vi "control-table.build.vi"(8 "error in (no error)":errorcluster, 11 "vi ref":refnum<vi>) -> (0 "error out":errorcluster, 3 "control table":string[][](array[string]), 5 "headers":string[](array[string])=["Label", "Caption", "Description", "Tip Strip"], 7 "control indicies":i32[](array[numeric]))   [LabVIEW 2020]
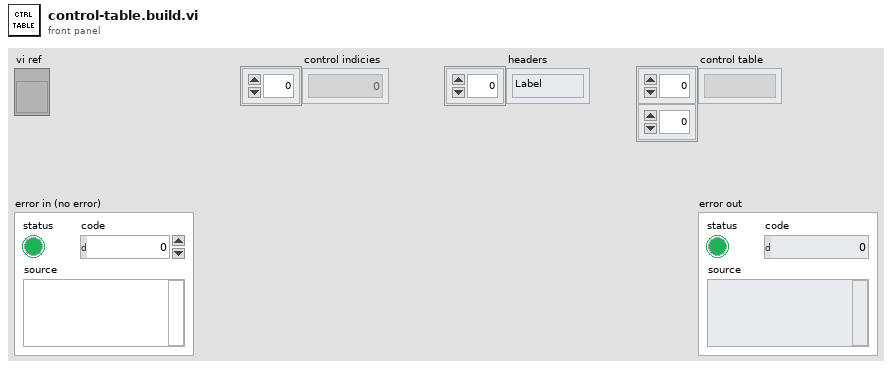
[diagram p1: front panel]
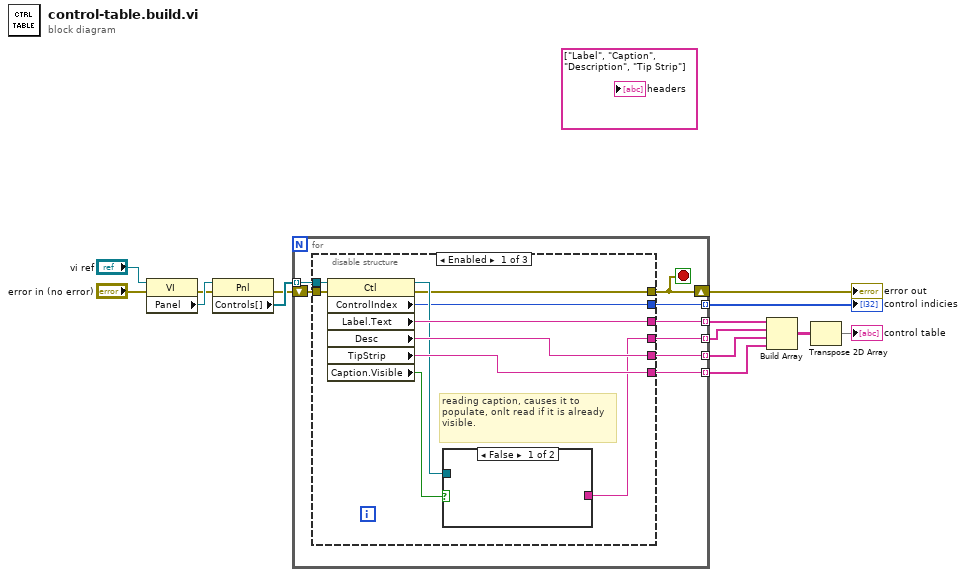
[diagram p0: block diagram]
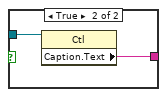
[diagram p2: hidden frame]
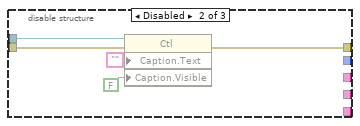
[diagram p3: hidden frame]
diagram:
  n1 = property class="VI"(reference="vi ref", error in="error in (no error)") -> (error out=w14:errorcluster, "Panel"=w15:refnum<vi>)  [unwired: 1 out]
  n2 = property class="Pnl"(reference=w15, error in=w14) -> (error out=w7:errorcluster, "Controls[]"=w13:refnum<vi>[])  [unwired: 1 out]
  n3 = for {
    tunnel: w13 -> [w23] mode=indexing
    tunnel: [w22] -> w12 mode=indexing
    tunnel: [w21] -> w11 mode=indexing
    tunnel: [w20] -> w10 mode=indexing
    tunnel: [w19] -> w8 mode=indexing
    shift-right: [w17] -> w2
    shift-left: w7 -> [w18]
    tunnel: [w16] -> w1 mode=indexing
    stop <- w17 stop-if-true
    n4 = disable-structure shown="Enabled" {
      disable-tunnel: w23 -> [w33 w40 _]
      disable-tunnel: [w32 _ _] -> w22
      disable-tunnel: [w31 _ _] -> w21
      disable-tunnel: [w30 _ _] -> w20
      disable-tunnel: [w27 _ _] -> w19
      disable-tunnel: w18 -> [w26 w39 w41]
      disable-tunnel: [w25 w38 w41] -> w17
      disable-tunnel: [w24 _ _] -> w16
      frame Enabled {
        # "reading caption, causes it to populate, onlt read if it is already visible."
        n5 = property class="Ctl"(reference=w33, error in=w26) -> (reference out=w29:refnum<vi>, error out=w25:errorcluster, "ControlIndex"=w24:i32, "Label.Text"=w32:string, "Desc"=w31:string, "TipStrip"=w30:string, "Caption.Visible"=w28:bool)
        n6 = case shown="False" w28 {
          tunnel: w29 -> [_ w35]
          tunnel: [_ w34] -> w27
          frame False {
          }
          frame True {
            n7 = property class="Ctl"(reference=w35) -> ("Caption.Text"=w34:string)  [unwired: 1 in, 2 out]
          }
        }
      }
      frame Disabled {
        n8 = property class="Ctl"(reference=w40, error in=w39, "Caption.Text"="", "Caption.Visible"=FALSE) -> (error out=w38:errorcluster)  [unwired: 1 out]
      }
      frame Disabled {
      }
    }
  }
  "error out" <- w2
  "control indicies" <- w1
  n9 = Build Array(w12, w8, w11, w10) -> (w9:string[][])
  n10 = Transpose 2D Array(2D array=w9) -> (transposed array=→"control table":string[][])
  "headers" <- string[] ["Label", "Caption", "Description", "Tip Strip"]
